vi "Excel Set Cell Format.vi"(0 "report in":refnum<class "NI_report.lvclass">, 5 "number format":string, 7 "start (-1, -1)":cluster{"row":i32, "column":i32}={"row"=-1, "column"=-1}, 9 "end (-1, -1)":cluster{"row":i32, "column":i32}={"row"=-1, "column"=-1}, 11 "error in (no error)":errorcluster, 12 "name (\"\")":string) -> (4 "report out":refnum<class "NI_report.lvclass">, 15 "error out":errorcluster)   [LabVIEW 2016, in "NI_Excel.lvclass"]
doc: "Sets the number format of the cells specified by the <B>start</B> and <B>end</B> clusters or by a named range."
uses:
  <vilib>/Utility/NIReport.llb/Excel/NI_Excel.lvclass
  <vilib>/Utility/NIReport.llb/NI_report.lvclass
  C:/Program Files (x86)/National Instruments/LabVIEW 2016/vi.lib/Utility/NIReport.llb/NI_report.lvclass
  <vilib>/Utility/NIReport.llb/Excel/NI_Excel.lvclass/NI_Excel.ctl
  <vilib>/addons/_office/NI_ReportGenerationToolkit.lvlib
  <vilib>/Utility/NIReport.llb/NI_ReportGenerationCore.lvlib
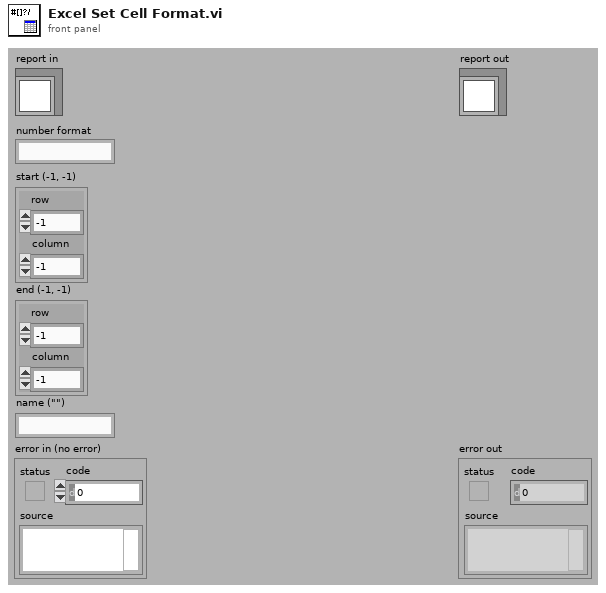
[diagram p1: front panel]
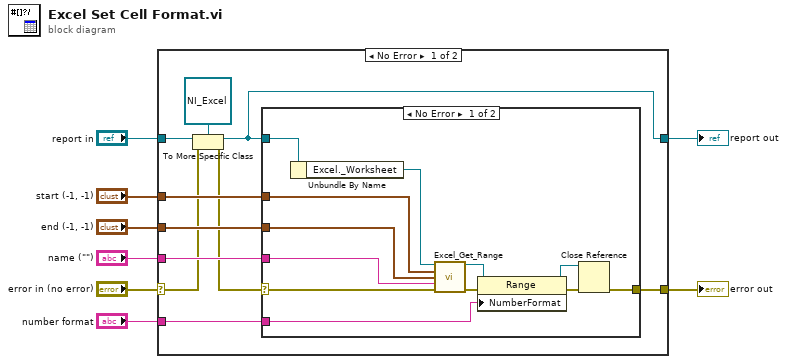
[diagram p0: block diagram]
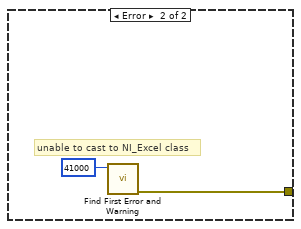
[diagram p2: hidden frame]
diagram:
  n1 = case shown="No Error" "error in (no error)" {
    selector: "error in (no error)" -> [w10 w34]
    tunnel: [w14 w34] -> w7
    tunnel: [w9 w33] -> w5
    tunnel: "report in" -> [w12 w33]
    tunnel: "start (-1, -1)" -> [w18 _]
    tunnel: "end (-1, -1)" -> [w17 _]
    tunnel: "name (\"\")" -> [w16 _]
    tunnel: "number format" -> [w15 _]
    frame No Error {
      n2 = To More Specific Class(target class=refnum<class "NI_Excel.lvclass"> refnum ("report in"), reference=w12, error in=w10) -> (specific class reference=w9:refnum<class "NI_Excel.lvclass">, error out=w11:errorcluster)
      n3 = case shown="No Error" w11 {
        selector: w11 -> [w19 _]
        tunnel: w18 -> [w27 _]
        tunnel: w17 -> [w26 _]
        tunnel: w16 -> [w25 _]
        tunnel: w15 -> [w24 _]
        tunnel: [w21 w31] -> w14
        tunnel: w9 -> [w20 _]
        frame No Error {
          n4 = Unbundle By Name(w20) -> ("Excel._Worksheet"=w29:refnum<k7>)
          n5 = call <vilib>:"Excel_Get_Range.vi"("Excel._Worksheet"=w29, "start"=w27, "end"=w26, "name"=w25, "error in (no error)"=w19) -> ("Range"=w23:refnum<k7>, "error out"=w30:errorcluster)  [unwired: 5 in, 4 out]
          n6 = property class="Range"(reference=w23, error in=w30, "NumberFormat"=w24) -> (reference out=w22:refnum<k7>, error out=w28:errorcluster)
          n7 = Close Reference(reference=w22, error in (no error)=w28) -> (error out=w21:errorcluster)
        }
        frame Error {
          # "unable to cast to NI_Excel class"
          n8 = call <vilib>:"Find First Error and Warning.vi"("error code"=41000) -> ("error out"=w31:errorcluster)  [unwired: 2 in, 4 out]
        }
      }
    }
    frame Error {
    }
  }
  "error out" <- w7
  "report out" <- w5
